vi "ListofImages(name,ext,size).vi"(10 "Folder Directory":string, 11 "Name of images":string[](array[string])) -> (3 "List of images (name, ext, size)":string[][](array[string]))   [LabVIEW 2020]
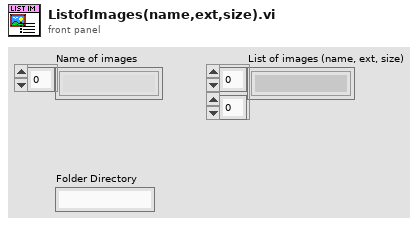
[diagram p1: front panel]
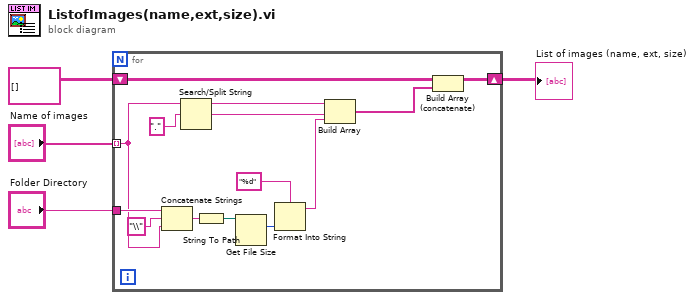
[diagram p0: block diagram]
diagram:
  n1 = for {
    tunnel: "Name of images" -> [w11] mode=indexing
    shift-right: [w13] -> w3
    shift-left: string[][] [] -> [w14]
    tunnel: "Folder Directory" -> [w12]
    n2 = Concatenate Strings(w12, "\\" ("string"), w11) -> (w9:string)
    n3 = Search/Split String(string=w11, search string/char (-)=".") -> (substring before match=w18:string, match + rest of string=w17:string)  [unwired: 1 in, 1 out]
    n4 = String To Path(string=w9) -> (path=w8:path)
    n5 = Get File Size(file=w8) -> (size (in bytes)=w7:i64)  [unwired: 1 in, 2 out]
    n6 = Format Into String(format string="%d", w7) -> (resulting string=w5:string)  [unwired: 2 in, 1 out]
    n7 = Build Array(w18, w17, w5) -> (w15:string[])
    n8 = Build Array (concatenate)(w14, w15) -> (w13:string[][])
  }
  "List of images (name, ext, size)" <- w3
